vi "z liveliness subscriber options default.vi"(8 "error in (no error)":errorcluster, 11 "this_":cluster{"history":bool}) -> (0 "error out":errorcluster, 3 "this_ out":cluster{"history":bool})   [LabVIEW 2021, in "zenohc.lvlib"]
doc: "void z_liveliness_subscriber_options_default(struct z_liveliness_subscriber_options_t *this_);"
uses:
  zenohc.lvlib
  zenohc.dll
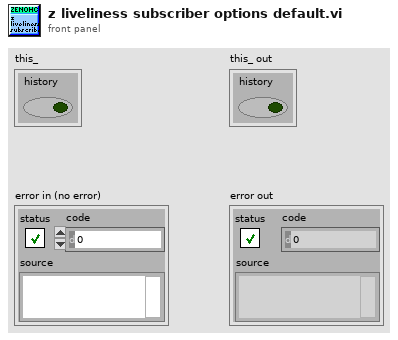
[diagram p1: front panel]
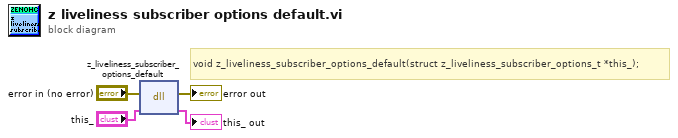
[diagram p0: block diagram]
diagram:
  # "void z_liveliness_subscriber_options_default(struct z_liveliness_subscriber_options_t *this_);"
  n1 = dll-call lib="D:/dev/zenoh_labview/zenohc/zenohc.*" fn="z_liveliness_subscriber_options_default"(error in="error in (no error)", "this_"="this_") -> (error out=→"error out":errorcluster, "this_"=→"this_ out":cluster{"history":bool})  [unwired: 3 in, 1 out]
